vi "from string.vi"(8 "error in":errorcluster, 9 "data":string, 10 "version":string, 11 "Standard Engine Repo Data in":refnum<class "Standard Engine Configuration.lvclass">) -> (0 "error out":errorcluster, 3 "Standard Engine Repo Data out":refnum<class "Standard Engine Configuration.lvclass">)   [LabVIEW 2013, in "Standard Engine Configuration.lvclass"]
uses:
  Standard Engine Configuration.lvclass
  timing policy.ctl
  <vilib>/NI/Module Execution Interface/Engine Configuration/engine configuration.lvclass
  Standard Engine Configuration.lvclass/Standard Engine Configuration.ctl
  Supported Timing Sources.ctl
  <vilib>/NI/Tag Bus Module Framework/runtime/error classification.ctl
  Error Actions.ctl
  Loop Info.ctl
  Module Specific Configuration.ctl
  Module Decimation.ctl
  Runtime/error responses.ctl
  error options.ctl
  <vilib>/NI/Configuration Framework/serializable configuration/NISE_CEF_serializable configuration.lvclass
  <vilib>/NI/Tag Bus Module Framework/runtime/TBM module execution interface.lvclass
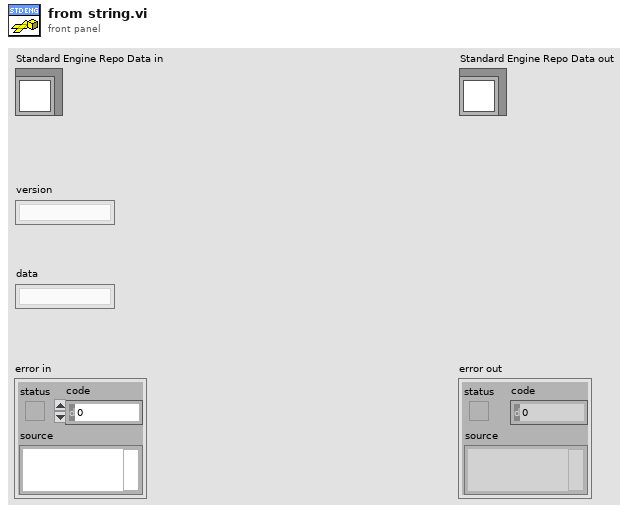
[diagram p1: front panel]
types:
  T1 = cluster{"Loop Info":cluster{"Processor":i32, "Priority":i32}, "Timing Source Type":enum16{"Use Module Timing Source", "1 kHz Clock", "1 MHz Clock", "Synchronize to Scan Engine"}, "Timing Source dt":u32, "Master Timing Module":string, "Module Specific Configuration":cluster{"Module ID":string, "Module Decimation":cluster{"Decimation":u16, "Offset":u16}, "Module Error Configuration":cluster{"Module Error Configuration":cluster{"error classification":enum16{"unknown", "none", "trivial", "recoverable", "critical"}, "Error Actions":enum16{"Clear", "Notify", "Stop Component", "Stop Engine", "Safe State", "Attempt Recovery"}[]}[]}, "execution order priority":i32, "async?":bool}[]}
  T2 = typedef "Standard Engine Configuration.lvclass/timing policy.ctl" = enum16{"strict determinism", "nonblocking", "nondeterministic inline"}
  T3 = typedef "Standard Engine Configuration.lvclass/Supported Timing Sources.ctl" = enum16{"Use Module Timing Source", "1 kHz Clock", "1 MHz Clock", "Synchronize to Scan Engine"}
  T4 = typedef "TBM module execution interface.lvclass/error classification.ctl" = enum16{"unknown", "none", "trivial", "recoverable", "critical"}
  T5 = typedef "Standard Engine Configuration.lvclass/Error Actions.ctl" = enum16{"Clear", "Notify", "Log", "Stop Component", "Stop Engine", "Safe State", "Attempt Recovery"}
  T6 = cluster{"Loop Info":cluster{"Processor":i32, "Priority":i32}, "Timing Source Type":T3, "Timing Source dt":u32, "Master Timing Module":string, "Module Specific Configuration":cluster{"Module ID":string, "Module Decimation":cluster{"Decimation":u16, "Offset":u16}, "Module Error Configuration":cluster{"Module Error Configuration":cluster{"error classification":T4, "Error Actions":T5[]}[]}, "execution order priority":i32, "async?":bool, "error tag":string}[]}
  T7 = typedef "Standard Engine Configuration.lvclass/Module Specific Configuration.ctl" = cluster{"Module ID":string, "Module Decimation":T8, "error tag":string, "error responses":T9}
  T8 = typedef "Standard Engine Configuration.lvclass/Module Decimation.ctl" = cluster{"Decimation":u16, "Offset":u16, "sort order":i32, "async?":bool}
  T9 = typedef "Standard Engine Configuration.lvclass/error responses.ctl" = cluster{"unknown":T10, "trivial":T10, "critical":T10, "recoverable":T10}
  T10 = typedef "Standard Engine Configuration.lvclass/error options.ctl" = cluster{"clear":bool, "notify":bool, "log":bool, "remove module":bool, "abort engine":bool, "go to safe state":bool, "recover module":bool}
  T11 = typedef "Standard Engine Configuration.lvclass/Loop Info.ctl" = cluster{"Processor":i32, "Priority":i32, "timing source type":T3, "module providing source":string, "timing source dt":u32, "timing policy":T2}
  T12 = typedef "Standard Engine Configuration.lvclass/Engine Configuration.ctl" = cluster{"Loop Info":T11, "Module Specific Configuration":T7[]}
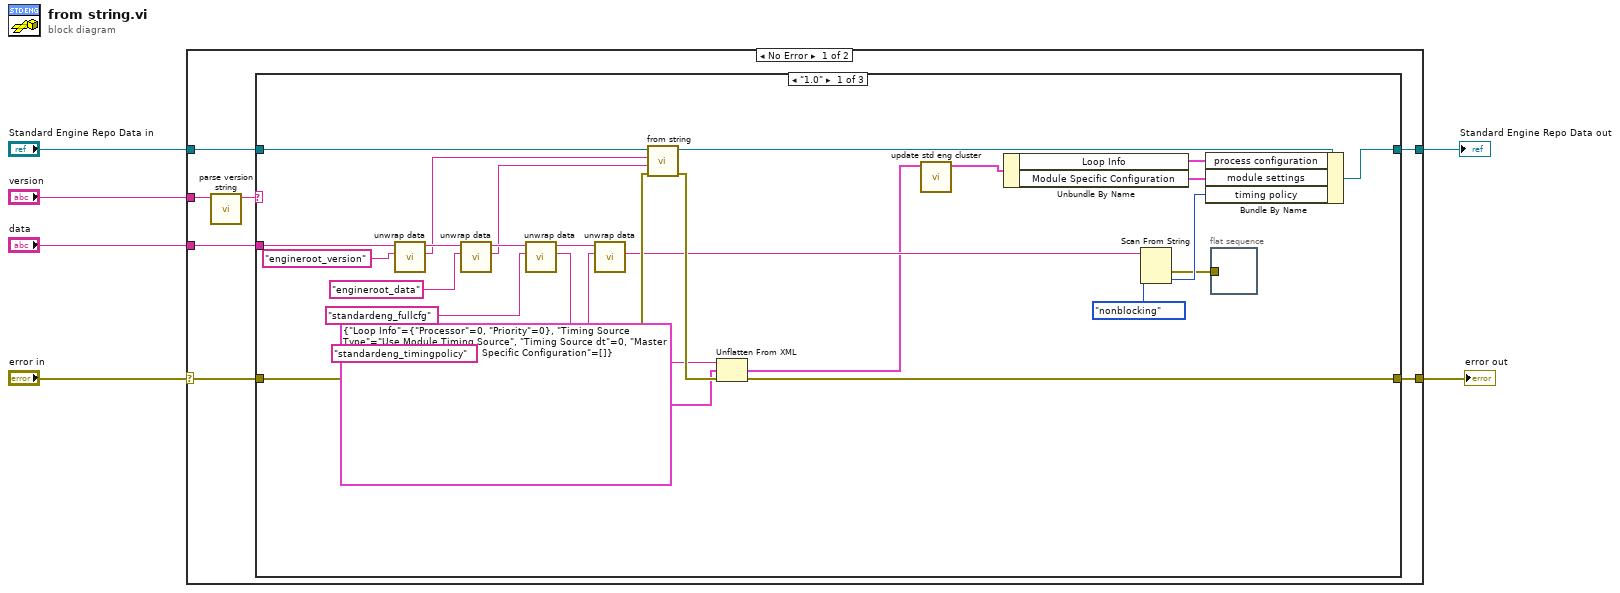
[diagram p0: block diagram]
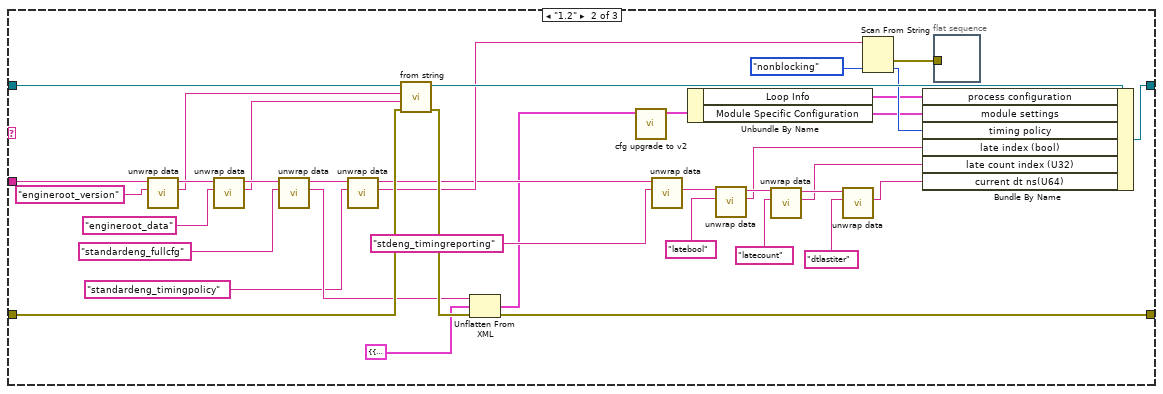
[diagram p2: hidden frame]
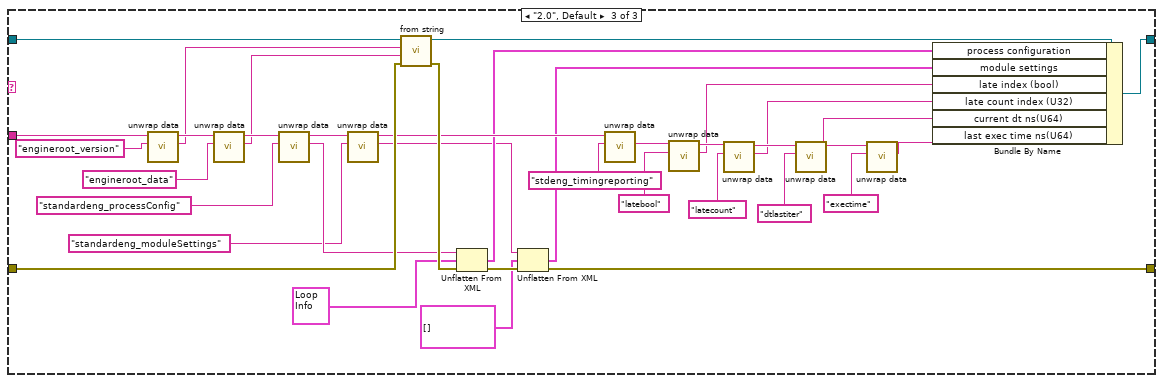
[diagram p3: hidden frame]
diagram:
  n1 = case shown="No Error" "error in" {
    selector: "error in" -> [w7 w114]
    tunnel: [w13 w114] -> w6
    tunnel: [w12 w115] -> w5
    tunnel: "data" -> [w11 _]
    tunnel: "Standard Engine Repo Data in" -> [w10 w115]
    tunnel: "version" -> [w9 _]
    frame No Error {
      n2 = call <vilib>:"parse version string.vi"("full version"=w9) -> ("major.minor version"=w8:string)  [unwired: 7 in, 3 out]
      n3 = case shown="\"1.0\"" w8 {
        tunnel: w7 -> [w39 w76 w113]
        tunnel: [w34 w71 w83] -> w13
        tunnel: [w37 w74 w111] -> w12
        tunnel: w11 -> [w28 w65 w102]
        tunnel: w10 -> [w36 w73 w110]
        frame "1.0" {
          n4 = call <vilib>:"unwrap data.vi"("identifier"="engineroot_version" ("additional identifier"), "data to unwrap"=w28) -> ("unwrapped data"=w27:string, "remaining string"=w29:string)  [unwired: 8 in]
          n5 = call <vilib>:"unwrap data.vi"("identifier"="engineroot_data" ("additional identifier"), "data to unwrap"=w29) -> ("unwrapped data"=w25:string, "remaining string"=w32:string)  [unwired: 8 in]
          n6 = call <vilib>:"unwrap data.vi"("identifier"="standardeng_fullcfg" ("additional identifier"), "data to unwrap"=w32) -> ("unwrapped data"=w26:string, "remaining string"=w24:string)  [unwired: 8 in]
          n7 = call <vilib>:"unwrap data.vi"("identifier"="standardeng_timingpolicy" ("additional identifier"), "data to unwrap"=w24) -> ("unwrapped data"=w22:string)  [unwired: 8 in, 1 out]
          n8 = call-parent "from string.vi"("error in"=w39, "data"=w25, "version"=w27, "engine configuration in"=w36) -> ("error out"=w38:errorcluster, "engine configuration out"=w35:refnum<class "Standard Engine Configuration.lvclass">)  [unwired: 6 in]
          n9 = Unflatten From XML(xml string=w26, type=T1 {"Loop Info"={"Processor"=0, "Priority"=0}, "Timing Source Type"=enum."Use Module Timing Source", "Timing Source dt"=0, "Master Timing Module"="", "Module Specific Configuration"=[]} ("Engine Configuration"), error in (no error)=w38) -> (value=w17:T1, error out=w34:errorcluster)
          n10 = call "update std eng cluster.vi"("Engine Configuration in"=w17) -> ("Engine Configuration out"=w14:T12)  [unwired: 10 in]
          n11 = Unbundle By Name(w14) -> ("Loop Info"=w16:T11, "Module Specific Configuration"=w15:T7[])
          n12 = Scan From String(input string=w22, default 1=timing_policy."nonblocking" ("timing policy")) -> (error out=w19:errorcluster, output 1=w20:T2)  [unwired: 3 in, 2 out]
          n13 = Bundle By Name(cluster=w35, "process configuration"=w16, "module settings"=w15, "timing policy"=w20) -> (w37:refnum<class "Standard Engine Configuration.lvclass">)
          n14 = flat-sequence {
            tunnel: w19 -> [_]
            frame #0 {
            }
          }
        }
        frame "1.2" {
          n15 = call <vilib>:"unwrap data.vi"("identifier"="engineroot_version" ("additional identifier"), "data to unwrap"=w65) -> ("unwrapped data"=w64:string, "remaining string"=w66:string)  [unwired: 8 in]
          n16 = call <vilib>:"unwrap data.vi"("identifier"="engineroot_data" ("additional identifier"), "data to unwrap"=w66) -> ("unwrapped data"=w62:string, "remaining string"=w69:string)  [unwired: 8 in]
          n17 = call <vilib>:"unwrap data.vi"("identifier"="standardeng_fullcfg" ("additional identifier"), "data to unwrap"=w69) -> ("unwrapped data"=w63:string, "remaining string"=w61:string)  [unwired: 8 in]
          n18 = call <vilib>:"unwrap data.vi"("identifier"="standardeng_timingpolicy" ("additional identifier"), "data to unwrap"=w61) -> ("unwrapped data"=w59:string, "remaining string"=w55:string)  [unwired: 8 in]
          n19 = call-parent "from string.vi"("error in"=w76, "data"=w62, "version"=w64, "engine configuration in"=w73) -> ("error out"=w75:errorcluster, "engine configuration out"=w72:refnum<class "Standard Engine Configuration.lvclass">)  [unwired: 6 in]
          n20 = Unflatten From XML(xml string=w63, type=T6 {"Loop Info"={"Processor"=-2, "Priority"=1}, "Timing Source Type"=enum."1 kHz Clock", "Timing Source dt"=5, "Master Timing Module"="", "Module Specific Configuration"=[]} ("Engine Configuration"), error in (no error)=w75) -> (value=w43:T6, error out=w71:errorcluster)
          n21 = call "cfg upgrade to v2.vi"("Engine Configuration"=w43) -> ("Engine Configuration out"=w42:T12)  [unwired: 10 in]
          n22 = call <vilib>:"unwrap data.vi"("identifier"="stdeng_timingreporting", "data to unwrap"=w55) -> ("unwrapped data"=w53:string)  [unwired: 8 in, 1 out]
          n23 = Unbundle By Name(w42) -> ("Loop Info"=w41:T11, "Module Specific Configuration"=w40:T7[])
          n24 = call <vilib>:"unwrap data.vi"("identifier"="latebool", "data to unwrap"=w53) -> ("unwrapped data"=w48:string, "remaining string"=w52:string)  [unwired: 8 in]
          n25 = call <vilib>:"unwrap data.vi"("identifier"="latecount", "data to unwrap"=w52) -> ("unwrapped data"=w49:string, "remaining string"=w51:string)  [unwired: 8 in]
          n26 = call <vilib>:"unwrap data.vi"("identifier"="dtlastiter", "data to unwrap"=w51) -> ("unwrapped data"=w50:string)  [unwired: 8 in, 1 out]
          n27 = Scan From String(input string=w59, default 1=timing_policy."nonblocking" ("timing policy")) -> (error out=w56:errorcluster, output 1=w57:T2)  [unwired: 3 in, 2 out]
          n28 = Bundle By Name(cluster=w72, "process configuration"=w41, "module settings"=w40, "timing policy"=w57, "late index (bool)"=w48, "late count index (U32)"=w49, "current dt ns(U64)"=w50) -> (w74:refnum<class "Standard Engine Configuration.lvclass">)
          n29 = flat-sequence {
            tunnel: w56 -> [_]
            frame #0 {
            }
          }
        }
        frame "2.0", Default {
          n30 = call <vilib>:"unwrap data.vi"("identifier"="engineroot_version" ("additional identifier"), "data to unwrap"=w102) -> ("unwrapped data"=w101:string, "remaining string"=w103:string)  [unwired: 8 in]
          n31 = call <vilib>:"unwrap data.vi"("identifier"="engineroot_data" ("additional identifier"), "data to unwrap"=w103) -> ("unwrapped data"=w99:string, "remaining string"=w106:string)  [unwired: 8 in]
          n32 = call <vilib>:"unwrap data.vi"("identifier"="standardeng_processConfig" ("additional identifier"), "data to unwrap"=w106) -> ("unwrapped data"=w100:string, "remaining string"=w98:string)  [unwired: 8 in]
          n33 = call <vilib>:"unwrap data.vi"("identifier"="standardeng_moduleSettings" ("additional identifier"), "data to unwrap"=w98) -> ("unwrapped data"=w80:string, "remaining string"=w96:string)  [unwired: 8 in]
          n34 = call-parent "from string.vi"("error in"=w113, "data"=w99, "version"=w101, "engine configuration in"=w110) -> ("error out"=w112:errorcluster, "engine configuration out"=w109:refnum<class "Standard Engine Configuration.lvclass">)  [unwired: 6 in]
          n35 = Unflatten From XML(xml string=w100, type=T11 {"Processor"=-2, "Priority"=1, "timing source type"=enum."1 MHz Clock", "module providing source"="", "timing source dt"=5000, "timing policy"=enum."nonblocking"} ("Loop Info"), error in (no error)=w112) -> (value=w84:T11, error out=w108:errorcluster)
          n36 = Unflatten From XML(xml string=w80, type=T7[] [] ("module settings"), error in (no error)=w108) -> (value=w81:T7[], error out=w83:errorcluster)
          n37 = call <vilib>:"unwrap data.vi"("identifier"="stdeng_timingreporting", "data to unwrap"=w96) -> ("unwrapped data"=w94:string)  [unwired: 8 in, 1 out]
          n38 = call <vilib>:"unwrap data.vi"("identifier"="latebool", "data to unwrap"=w94) -> ("unwrapped data"=w89:string, "remaining string"=w93:string)  [unwired: 8 in]
          n39 = call <vilib>:"unwrap data.vi"("identifier"="latecount", "data to unwrap"=w93) -> ("unwrapped data"=w90:string, "remaining string"=w92:string)  [unwired: 8 in]
          n40 = call <vilib>:"unwrap data.vi"("identifier"="dtlastiter", "data to unwrap"=w92) -> ("unwrapped data"=w91:string, "remaining string"=w78:string)  [unwired: 8 in]
          n41 = call <vilib>:"unwrap data.vi"("identifier"="exectime", "data to unwrap"=w78) -> ("unwrapped data"=w79:string)  [unwired: 8 in, 1 out]
          n42 = Bundle By Name(cluster=w109, "process configuration"=w84, "module settings"=w81, "late index (bool)"=w89, "late count index (U32)"=w90, "current dt ns(U64)"=w91, "last exec time ns(U64)"=w79) -> (w111:refnum<class "Standard Engine Configuration.lvclass">)
        }
      }
    }
    frame Error {
    }
  }
  "error out" <- w6
  "Standard Engine Repo Data out" <- w5
